vi "AndorMISSINGPARTS.vi"   [LabVIEW 2018, in "AndorOWN.lvlib"]
uses:
  AndorOWN.lvlib
  <userlib>/Andor SDK/Andor SDK.lvlib
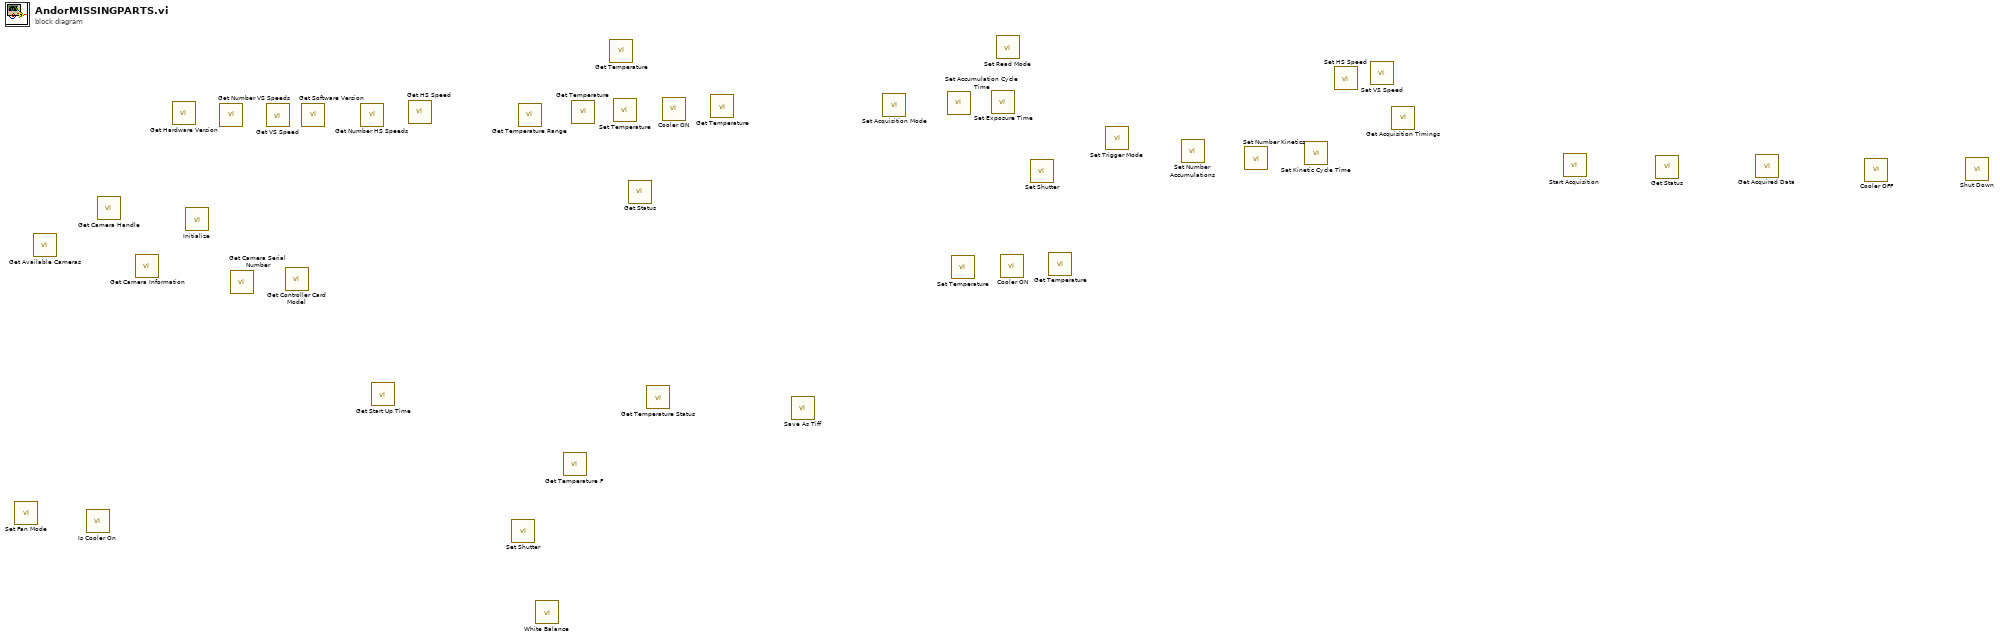
[diagram p0: block diagram]
diagram:
  n1 = call <userlib>:"Set Fan Mode.vi"() -> ()  [unwired: 11 in, 1 out]
  n2 = call <userlib>:"Get Available Cameras.vi"() -> ()  [unwired: 10 in, 2 out]
  n3 = call <userlib>:"Is Cooler On.vi"() -> ()  [unwired: 10 in, 2 out]
  n4 = call <userlib>:"Get Camera Handle.vi"() -> ()  [unwired: 10 in, 2 out]
  n5 = call <userlib>:"Get Camera Information.vi"() -> ()  [unwired: 10 in, 2 out]
  n6 = call <userlib>:"Get Hardware Version.vi"() -> ()  [unwired: 9 in, 7 out]
  n7 = call <userlib>:"Initialize.vi"() -> ()  [unwired: 10 in, 2 out]
  n8 = call <userlib>:"Get Number VS Speeds.vi"() -> ()  [unwired: 10 in, 2 out]
  n9 = call <userlib>:"Get Camera Serial Number.vi"() -> ()  [unwired: 9 in, 3 out]
  n10 = call <userlib>:"Get VS Speed.vi"() -> ()  [unwired: 10 in, 2 out]
  n11 = call <userlib>:"Get Controller Card Model.vi"() -> ()  [unwired: 9 in, 3 out]
  n12 = call <userlib>:"Get Software Version.vi"() -> ()  [unwired: 9 in, 7 out]
  n13 = call <userlib>:"Get Number HS Speeds.vi"() -> ()  [unwired: 10 in, 2 out]
  n14 = call <userlib>:"Get Start Up Time.vi"() -> ()  [unwired: 10 in, 2 out]
  n15 = call <userlib>:"Get HS Speed.vi"() -> ()  [unwired: 10 in, 2 out]
  n16 = call <userlib>:"Set Shutter.vi"() -> ()  [unwired: 11 in, 1 out]
  n17 = call <userlib>:"Get Temperature Range.vi"() -> ()  [unwired: 9 in, 3 out]
  n18 = call <userlib>:"White Balance.vi"() -> ()  [unwired: 9 in, 7 out]
  n19 = call <userlib>:"Get Temperature F.vi"() -> ()  [unwired: 10 in, 2 out]
  n20 = call <userlib>:"Get Temperature.vi"() -> ()  [unwired: 10 in, 2 out]
  n21 = call <userlib>:"Get Temperature.vi"() -> ()  [unwired: 10 in, 2 out]
  n22 = call <userlib>:"Set Temperature.vi"() -> ()  [unwired: 11 in, 1 out]
  n23 = call <userlib>:"Get Status.vi"() -> ()  [unwired: 10 in, 2 out]
  n24 = call <userlib>:"Get Temperature Status.vi"() -> ()  [unwired: 7 in, 5 out]
  n25 = call <userlib>:"Cooler ON.vi"() -> ()  [unwired: 11 in, 1 out]
  n26 = call <userlib>:"Get Temperature.vi"() -> ()  [unwired: 10 in, 2 out]
  n27 = call <userlib>:"Save As Tiff.vi"() -> ()  [unwired: 9 in, 3 out]
  n28 = call <userlib>:"Set Acquisition Mode.vi"() -> ()  [unwired: 11 in, 1 out]
  n29 = call <userlib>:"Set Accumulation Cycle Time.vi"() -> ()  [unwired: 11 in, 1 out]
  n30 = call <userlib>:"Set Temperature.vi"() -> ()  [unwired: 11 in, 1 out]
  n31 = call <userlib>:"Set Exposure Time.vi"() -> ()  [unwired: 11 in, 1 out]
  n32 = call <userlib>:"Set Read Mode.vi"() -> ()  [unwired: 11 in, 1 out]
  n33 = call <userlib>:"Cooler ON.vi"() -> ()  [unwired: 11 in, 1 out]
  n34 = call <userlib>:"Set Shutter.vi"() -> ()  [unwired: 11 in, 1 out]
  n35 = call <userlib>:"Get Temperature.vi"() -> ()  [unwired: 10 in, 2 out]
  n36 = call <userlib>:"Set Trigger Mode.vi"() -> ()  [unwired: 11 in, 1 out]
  n37 = call <userlib>:"Set Number Accumulations.vi"() -> ()  [unwired: 11 in, 1 out]
  n38 = call <userlib>:"Set Number Kinetics.vi"() -> ()  [unwired: 11 in, 1 out]
  n39 = call <userlib>:"Set Kinetic Cycle Time.vi"() -> ()  [unwired: 11 in, 1 out]
  n40 = call <userlib>:"Set HS Speed.vi"() -> ()  [unwired: 11 in, 1 out]
  n41 = call <userlib>:"Set VS Speed.vi"() -> ()  [unwired: 11 in, 1 out]
  n42 = call <userlib>:"Get Acquisition Timings.vi"() -> ()  [unwired: 8 in, 4 out]
  n43 = call <userlib>:"Start Acquisition.vi"() -> ()  [unwired: 11 in, 1 out]
  n44 = call <userlib>:"Get Status.vi"() -> ()  [unwired: 10 in, 2 out]
  n45 = call <userlib>:"Get Acquired Data.vi"() -> ()  [unwired: 10 in, 2 out]
  n46 = call <userlib>:"Cooler OFF.vi"() -> ()  [unwired: 11 in, 1 out]
  n47 = call <userlib>:"Shut Down.vi"() -> ()  [unwired: 11 in, 1 out]
